vi "is directory.vi"(1 "Path":path) -> (0 "Does the path point to a directory (a folder)?":bool)   [LabVIEW 2022 SP3]
doc: "This VI returns True if and only if the input path points to a folder (not a file)."
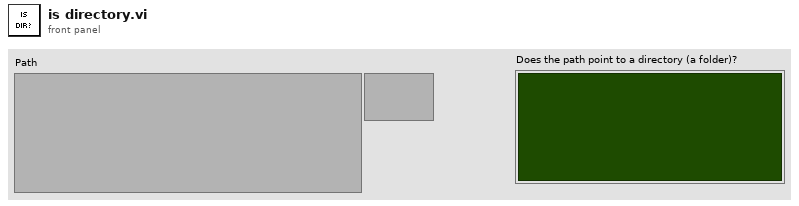
[diagram p1: front panel]
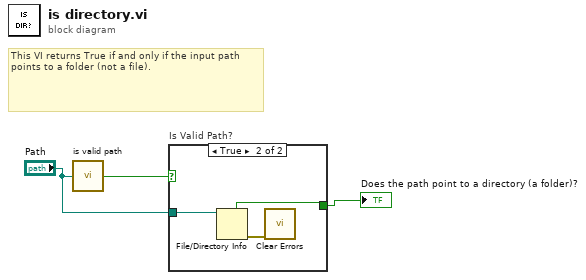
[diagram p0: block diagram]
diagram:
  # "This VI returns True if and only if the input path points to a folder (not a file)."
  n1 = call "is valid path.vi"("Path"="Path") -> ("Is valid path?"=w1:bool)
  n2 = case "Is Valid Path?" shown="True" w1 {
    tunnel: [_ w6] -> w3
    tunnel: "Path" -> [_ w5]
    frame False {
    }
    frame True {
      n3 = File/Directory Info(path=w5) -> (directory=w6:bool, error out=w4:errorcluster)  [unwired: 1 in, 5 out]
      n4 = call <vilib>:"Clear Errors.vi"("error in (no error)"=w4) -> ()  [unwired: 5 in, 2 out]
    }
  }
  "Does the path point to a directory (a folder)?" <- w3
